vi "Error Action Loader.vi"(6 "First Call?":bool, 8 "error in (no error)":errorcluster, 11 "LAC Error Logger in":refnum<class "LAC Error Logger.lvclass">) -> (0 "error out":errorcluster, 3 "LAC Error Logger out":refnum<class "LAC Error Logger.lvclass">)   [LabVIEW 2017, in "Assert API Components.lvlib" / "Log Assert Core.lvlib" / "LAC Error Logger.lvclass"]
uses:
  LAC Error Logger.lvclass
  Error File/Error File.lvclass
  C:/Users/ukhornp/Documents/Work/Projects/actor_assert_api/Core/Assert API Components/Log Assert Core Components/LAC Error Logger/LAC Error Logger.lvclass
  Debug UI/Debug UI.lvclass
  <vilib>/Utility/config.llb/Read Key (String).vi
  Assert API Components.lvlib
  <vilib>/Utility/config.llb/NI_LVConfig.lvlib
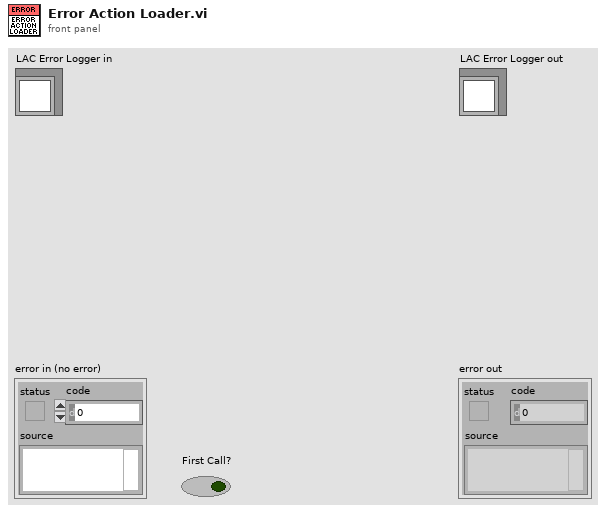
[diagram p1: front panel]
types:
  T1 = typedef "NI_LVConfig.lvlib/Config Data RefNum.ctl" = refnum<k1>
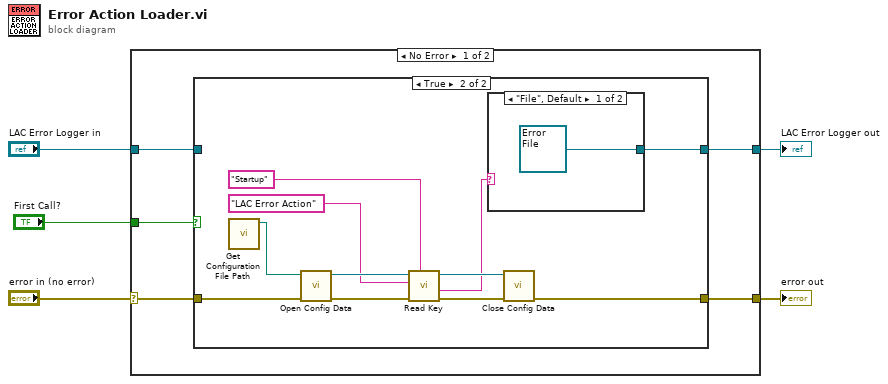
[diagram p0: block diagram]
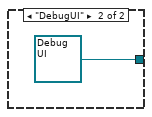
[diagram p3: hidden frame]
diagram:
  n1 = case shown="No Error" "error in (no error)" {
    selector: "error in (no error)" -> [w7 w27]
    tunnel: [w6 w27] -> w4
    tunnel: [w8 w26] -> w2
    tunnel: "LAC Error Logger in" -> [w9 w26]
    tunnel: "First Call?" -> [w10 _]
    frame No Error {
      n2 = case shown="True" w10 {
        tunnel: w9 -> [w12 _]
        tunnel: [w12 w13] -> w8
        tunnel: w7 -> [w11 w19]
        tunnel: [w11 w18] -> w6
        frame False {
        }
        frame True {
          n3 = call "Get Configuration File Path.vi"() -> ("Configuration File Path"=w15:path)  [unwired: 11 in]
          n4 = call <vilib>:"Open Config Data.vi"("error in (no error)"=w19, "configuration file path"=w15) -> ("error out"=w22:errorcluster, "refnum"=w23:T1)  [unwired: 7 in, 1 out]
          n5 = call-poly <vilib>:"Read Key.vi"("section"="Startup", "error in (no error)"=w22, "key"="LAC Error Action", "refnum"=w23) -> ("error out"=w20:errorcluster, "value"=w14:string, "refnum out"=w21:T1)  [unwired: 4 in, 1 out]
          n6 = case shown="\"File\", Default" w14 {
            tunnel: [refnum<class "Error File.lvclass"> refnum ("Assert API Components.lvlib:Log Assert Core.lvlib:Error File.lvclass") refnum<class "Debug UI.lvclass"> refnum ("Assert API Components.lvlib:Log Assert Core.lvlib:Debug UI.lvclass")] -> w13
            frame "File", Default {
            }
            frame "DebugUI" {
            }
          }
          n7 = call <vilib>:"Close Config Data.vi"("error in (no error)"=w20, "refnum"=w21) -> ("error out"=w18:errorcluster)  [unwired: 8 in, 1 out]
        }
      }
    }
    frame Error {
    }
  }
  "error out" <- w4
  "LAC Error Logger out" <- w2
